vi "ADIS16470 Loop.vi"(8 "error in":errorcluster) -> ()   [LabVIEW 2019]
uses:
  Typedef/ADIS16470 Device Reference.ctl
  Typedef/ADIS16470 Hardware Configuration.ctl
  <vilib>/Rock Robotics/WPI/SPI/WPI_SPIMode.ctl
  <vilib>/Rock Robotics/SystemInterfaces/DIO/FPGA_DIOChannel.ctl
  <vilib>/Rock Robotics/SystemInterfaces/spilib/spi_bus.ctl
  Typedef/ADIS16470 Status.ctl
  Typedef/ADIS16470 Data.ctl
  Typedef/ADIS16470 Process.ctl
  Typedef/ADIS16470 Command Type.ctl
  <vilib>/Rock Robotics/SystemInterfaces/CounterEncoderSourceConvertion/FPGA_CounterEncoderSourceConvertionLVSourceType.ctl
  <vilib>/Rock Robotics/SystemInterfaces/DIO/FPGA_DIODigitalSourceChannel.ctl
  <vilib>/Rock Robotics/SystemInterfaces/AnalogTrigger/FPGA_AnalogTriggerIndex.ctl
  <vilib>/Rock Robotics/SystemInterfaces/AnalogTrigger/FPGA_AnalogTriggerOutType.ctl
  Typedef/ADIS16470 Calibration Time.ctl
  <vilib>/Rock Robotics/WPI/SPI/WPI_SPIDevRef.ctl
  Typedef/ADIS16470 Register.ctl
  <vilib>/Rock Robotics/WPI/Counter/WPI_CounterDigitalInputToDigitalSource.vi
panel:
  in  "Calibration Time":T1
  in  "element":T2
  out "Waveform Chart":dbl(graph)
  out "Offset Bias":i16[](array[numeric])
  in  "ADIS16470DevRef":T3={"DevStatus"={"status"=FALSE, "code"=0, "source"=""}, "Hardware Config"={"SPI Clock Rate (Hz)"=1000000.0, "IMU SPI Mode (3)"=enum."Mode 3 (Clk Idle High,Sample on Trailing)", "IMU Reset Pin"=enum."SPI Port CS2", "IMU SPI Bus"=enum."SPI On-Board, CS0", "IMU Data Ready Pin"=enum."SPI Port CS1", "Stall Config"={"Pow2BytesPerRead"=255, "StallTicks"=640, "CsToSclkTicks"=5}}, "Calibration Complete"=refnum, "Status FIFO"=refnum, "Last Value Reference"=refnum, "Sychronous Process VI"=refnum, "Cmd FIFO"=refnum, "Source"={"DevStatus"={"status"=FALSE, "code"=0, "source"=""}, "AnalogTriggerMode?"=FALSE, "DigitalMode"={"DIO Channel"=enum."Disabled"}, "AnalogTriggerMode"={"AnalogTriggerIndex"=enum."Trig 0", "OutputType"=enum."InWindow"}}, "Data FIFO"=refnum, "Calibration Time"=enum."1s"}
  in  "Main Name":string
  # "XG_BIAS_LOW"
  # "XG_BIAS_HIGH"
  # "YG_BIAS_LOW"
  # "YG_BIAS_HIGH"
  # "ZG_BIAS_LOW"
  # "ZG_BIAS_HIGH"
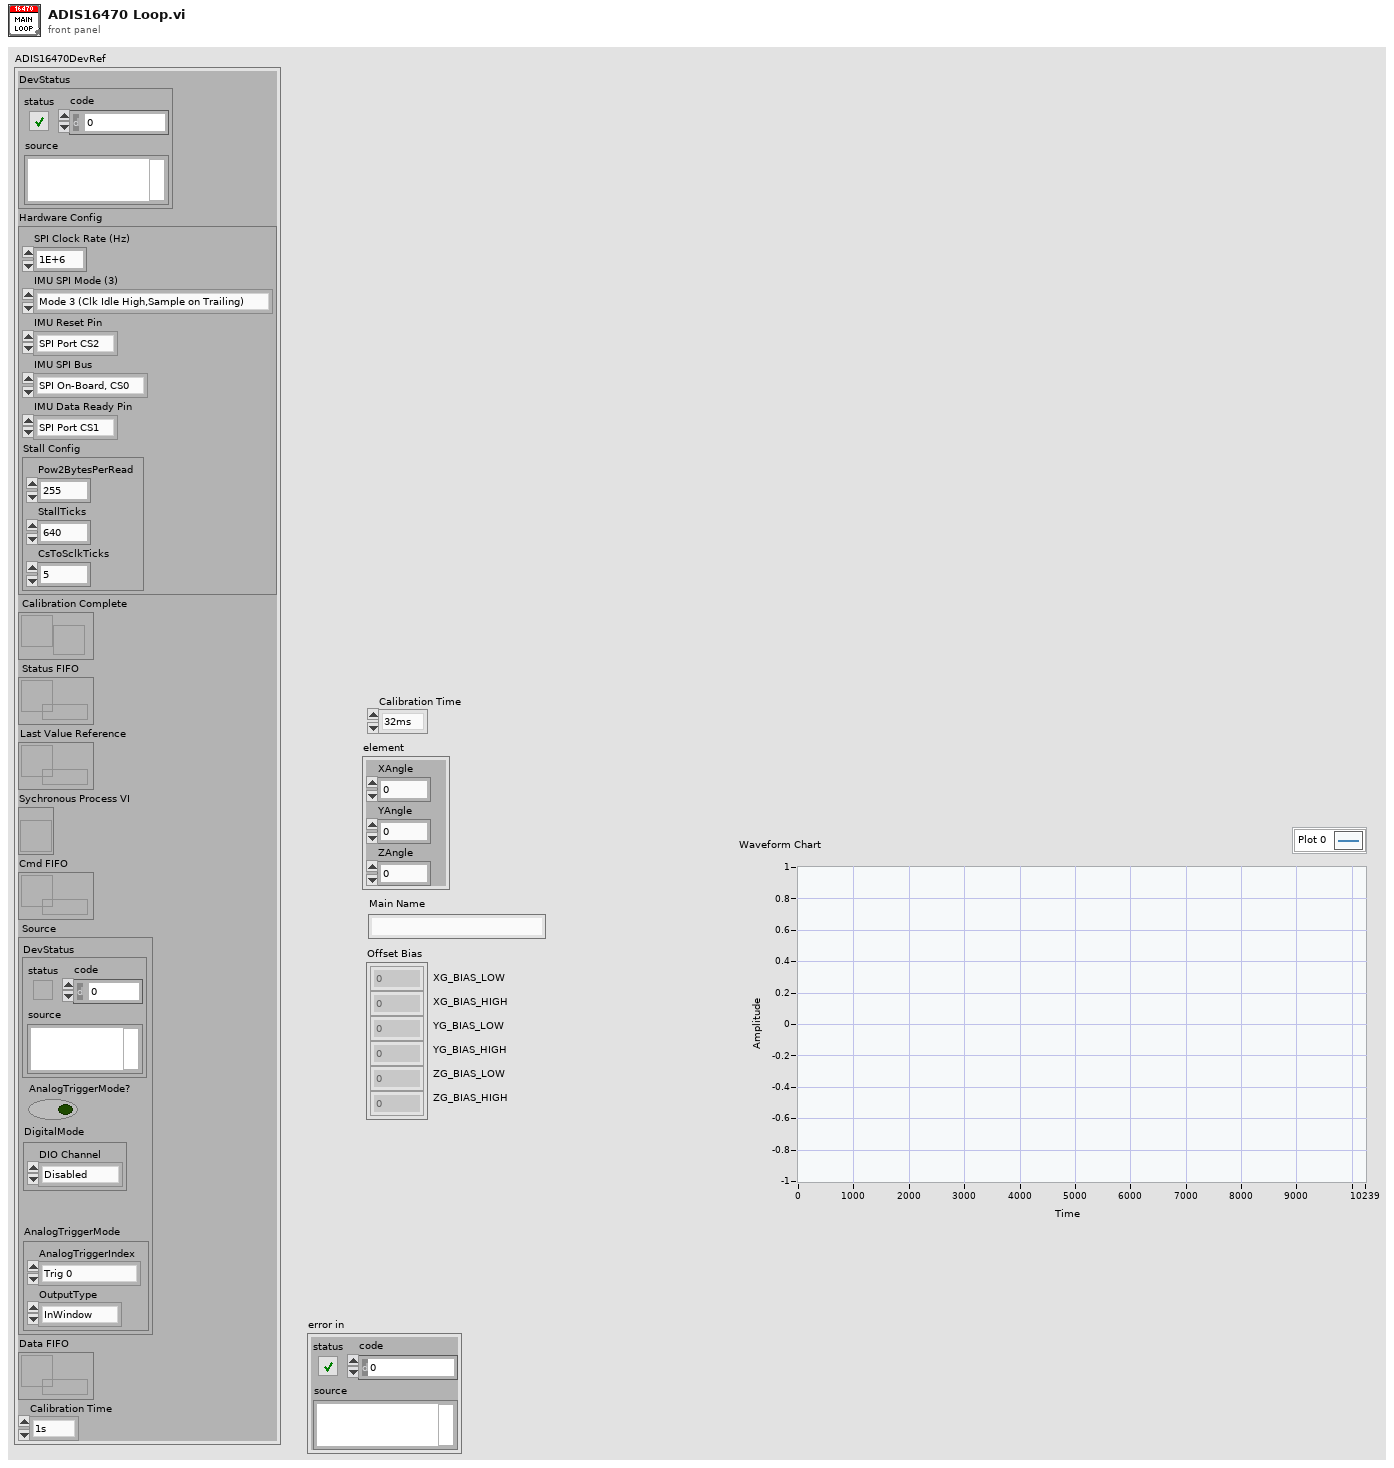
[diagram p1: front panel]
types:
  T1 = typedef "ADIS16470 Calibration Time.ctl" = enum16{"32ms", "64ms", "128ms", "256ms", "512ms", "1s", "2s", "4s", "8s", "16s", "32s", "64s"}
  T2 = typedef "ADIS16470 Data.ctl" = cluster{"XAngle":dbl, "YAngle":dbl, "ZAngle":dbl}
  T3 = typedef "ADIS16470 Device Reference.ctl" = cluster{"DevStatus":errorcluster, "Hardware Config":T4, "Calibration Complete":refnum<notifier>, "Status FIFO":refnum<k33>, "Last Value Reference":refnum<data-value>, "Sychronous Process VI":T8, "Cmd FIFO":refnum<k33>, "Source":T9, "Data FIFO":refnum<k33>, "Calibration Time":T1}
  T4 = typedef "ADIS16470 Hardware Configuration.ctl" = cluster{"SPI Clock Rate (Hz)":dbl, "IMU SPI Mode (3)":T5, "IMU Reset Pin":T6, "IMU SPI Bus":T7, "IMU Data Ready Pin":T6, "Stall Config":cluster{"Pow2BytesPerRead":u8, "StallTicks":u16, "CsToSclkTicks":u8}}
  T5 = typedef "WPI_SPIMode.ctl" = enum16{"Mode 0 (Clk Idle Low,Sample on Leading)", "Mode 1 (Clk Idle Low,Sample on Trailing)", "Mode 2 (Clk Idle High,Sample on Leading)", "Mode 3 (Clk Idle High,Sample on Trailing)"}
  T6 = typedef "FPGA_DIOChannel.ctl" = enum8{"DIO 0", "DIO 1", "DIO 2", "DIO 3", "DIO 4", "DIO 5", "DIO 6", "DIO 7", "DIO 8", "DIO 9", "DIO MXP 0", "DIO MXP 1", "DIO MXP 2", "DIO MXP 3", "DIO MXP 4", "DIO MXP 5", "DIO MXP 6", "DIO MXP 7", "DIO MXP 8", "DIO MXP 9", "DIO MXP 10", "DIO MXP 11", "DIO MXP 12", "DIO MXP 13", "DIO MXP 14", "DIO MXP 15", "SPI Port CS1", "SPI Port CS2", "SPI Port CS3", "SPI Port MISO", "SPI Port MOSI", "Invalid"}
  T7 = typedef "spi_bus.ctl" = enum16{"SPI On-Board, CS0", "SPI On-Board, CS1", "SPI On-Board, CS2", "SPI On-Board, CS3", "SPI MXP", "Invalid"}
  T8 = typedef "ADIS16470 Process.ctl" = refnum<vi>
  T9 = typedef "FPGA_CounterEncoderSourceConvertionLVSourceType.ctl" = cluster{"DevStatus":errorcluster, "AnalogTriggerMode?":bool, "DigitalMode":cluster{"DIO Channel":T10}, "AnalogTriggerMode":cluster{"AnalogTriggerIndex":T11, "OutputType":T12}}
  T10 = typedef "FPGA_DIODigitalSourceChannel.ctl" = enum8{"DIO 0", "DIO 1", "DIO 2", "DIO 3", "DIO 4", "DIO 5", "DIO 6", "DIO 7", "DIO 8", "DIO 9", "DIO MXP 0", "DIO MXP 1", "DIO MXP 2", "DIO MXP 3", "DIO MXP 4", "DIO MXP 5", "DIO MXP 6", "DIO MXP 7", "DIO MXP 8", "DIO MXP 9", "DIO MXP 10", "DIO MXP 11", "DIO MXP 12", "DIO MXP 13", "DIO MXP 14", "DIO MXP 15", "SPI Port CS1", "SPI Port CS2", "SPI Port CS3", "SPI Port MISO", "SPI Port MOSI", "Disabled"}
  T11 = typedef "FPGA_AnalogTriggerIndex.ctl" = enum8{"Trig 0", "Trig 1", "Trig 2", "Trig 3", "Trig 4", "Trig 5", "Trig 6", "Trig 7", "Invalid"}
  T12 = typedef "FPGA_AnalogTriggerOutType.ctl" = enum16{"InWindow", "TriggerState", "Rising", "Falling"}
  T13 = typedef "WPI_SPIDevRef.ctl" = cluster{"DevStatus":errorcluster, "Handle":i32, "SPI Bus":T7}
  T14 = typedef "ADIS16470 Register.ctl" = u8
  T15 = cluster{"SPIDevRef":T13, "Data Counter":u16, "Reset":bool, "Digital Source":T9, "Bytes Per Sample":u32, "Data":dbl[], "ADIS16470DevRef":T3, "TimeStampPrev":u32, "Sensor to Robot Rotation":dbl[][], "Data Packet":T14[], "AutoSPI Active?":bool}
  T16 = typedef "ADIS16470 Status.ctl" = cluster{"Calibrated?":bool, "IMU Detected?":bool}
  T17 = typedef "ADIS16470 Command Type.ctl" = cluster{"Command":enum16{"None", "Reset", "Set Calibration Period", "Recalibrate", "Recal Complete", "Exit Auto SPI", "Start Auto SPI"}, "Data":u32}
  T18 = typedef "WPI_DigitalOutputDevRef.ctl" = cluster{"DIO Channel":T6, "DevStatus":errorcluster}
  T19 = typedef "WPI_DigitalInputDevRef.ctl" = cluster{"DevStatus":errorcluster, "DIO Channel":T6}
  T20 = cluster{"Pow2BytesPerRead":u8, "StallTicks":u16, "CsToSclkTicks":u8}
  T21 = enum16{"None", "Reset", "Set Calibration Period", "Recalibrate", "Recal Complete", "Exit Auto SPI", "Start Auto SPI"}
  T22 = enum32{"Bad", "Idle", "Run top level", "Running"}
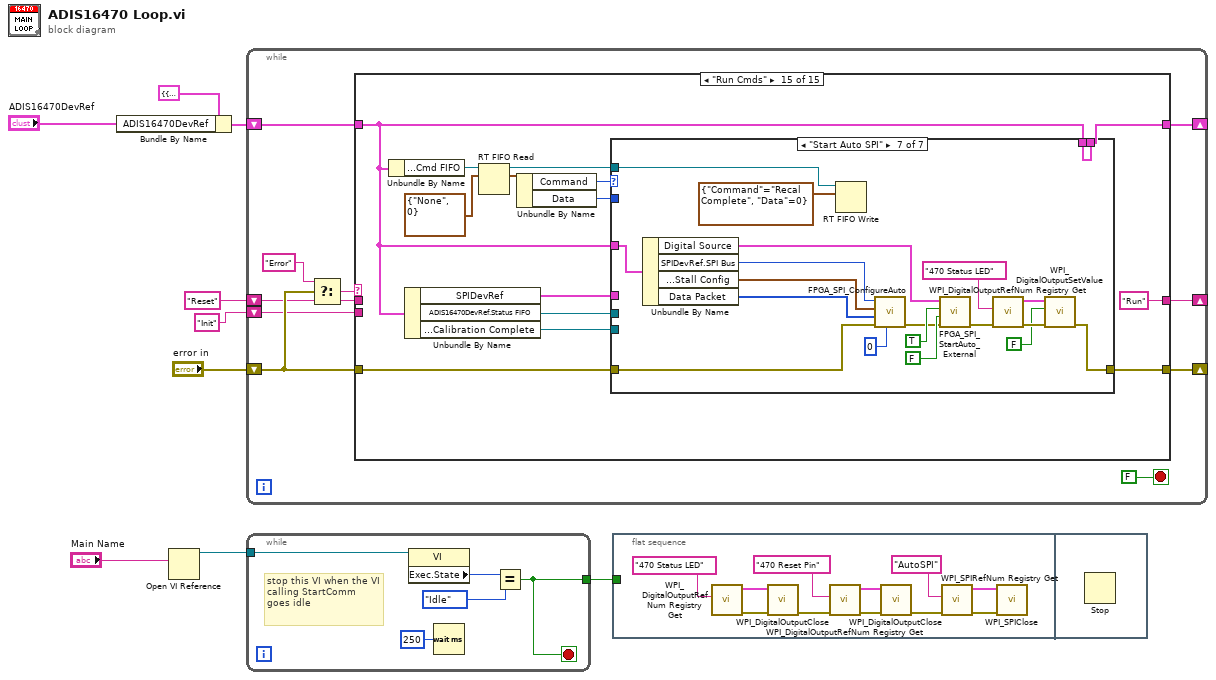
[diagram p0: block diagram]
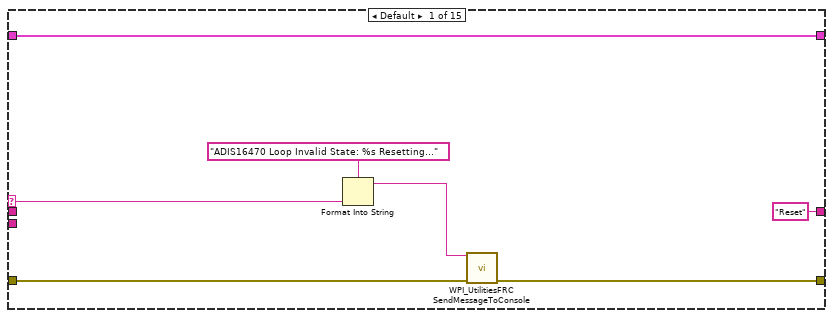
[diagram p2: hidden frame]
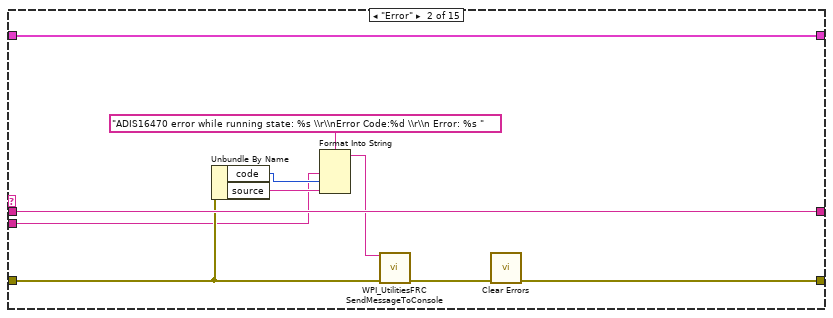
[diagram p3: hidden frame]
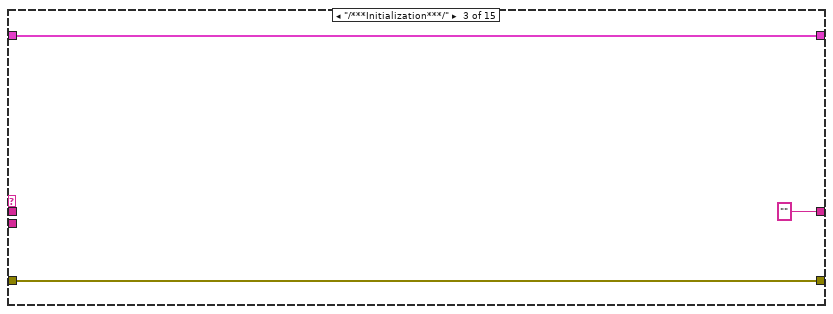
[diagram p4: hidden frame]
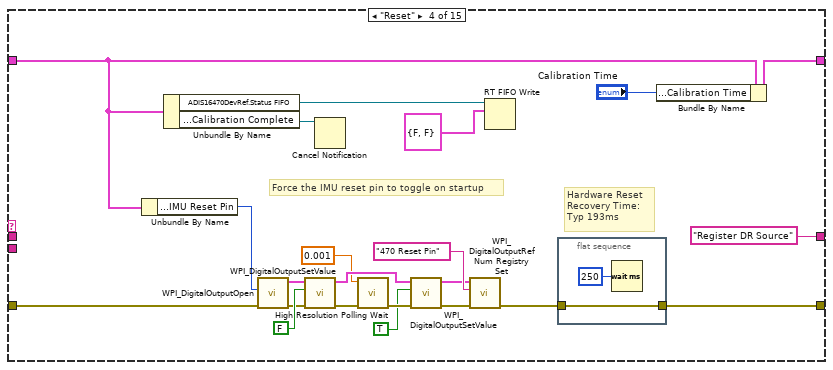
[diagram p5: hidden frame]
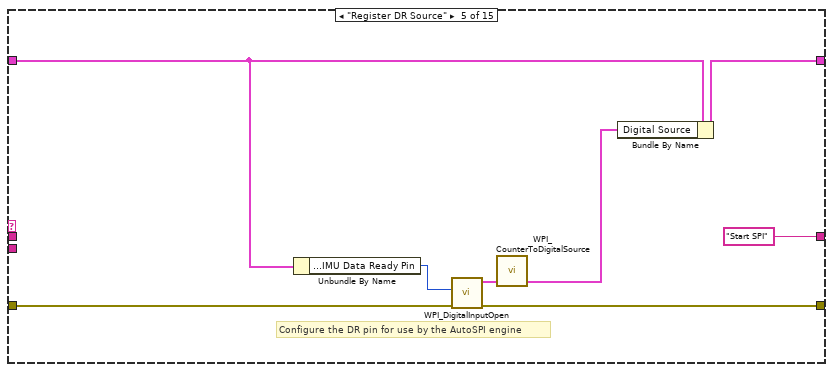
[diagram p6: hidden frame]
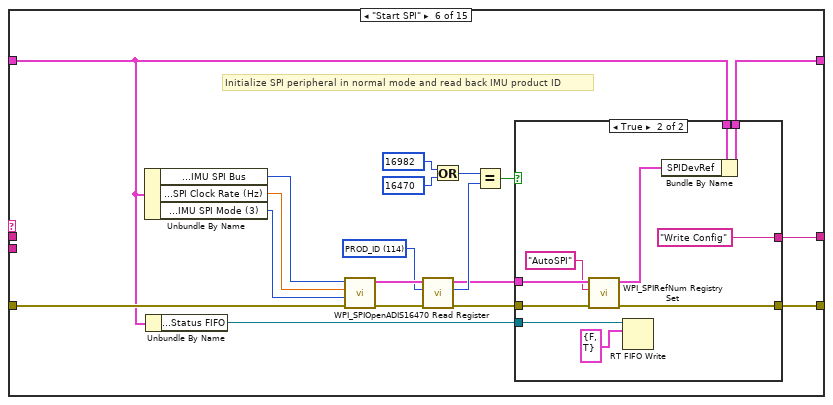
[diagram p7: hidden frame]
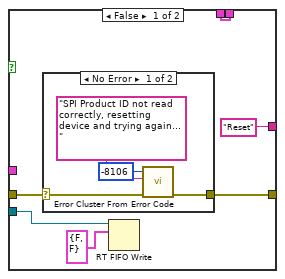
[diagram p8: hidden frame]
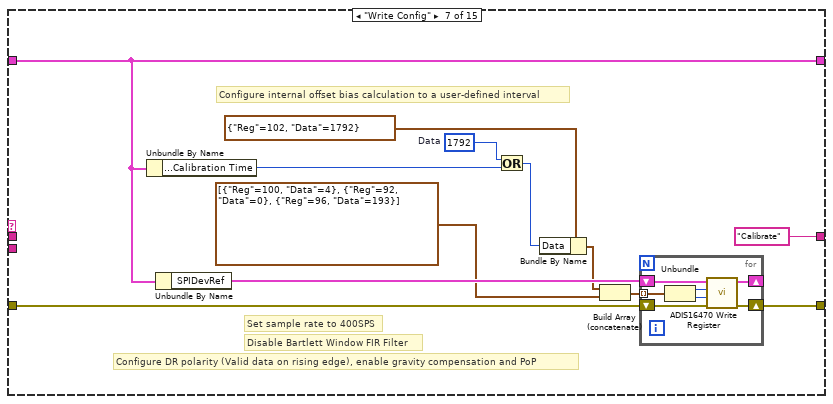
[diagram p10: hidden frame]
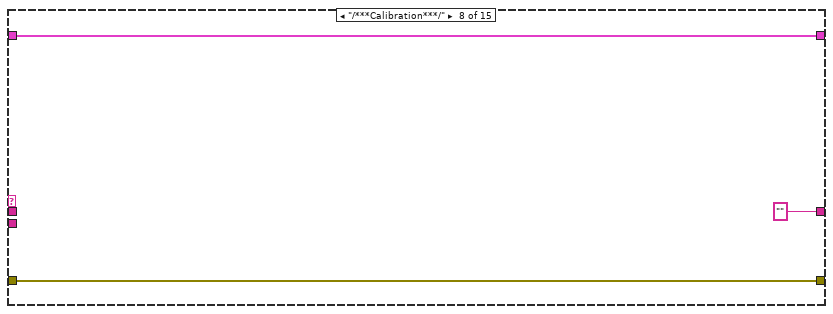
[diagram p11: hidden frame]
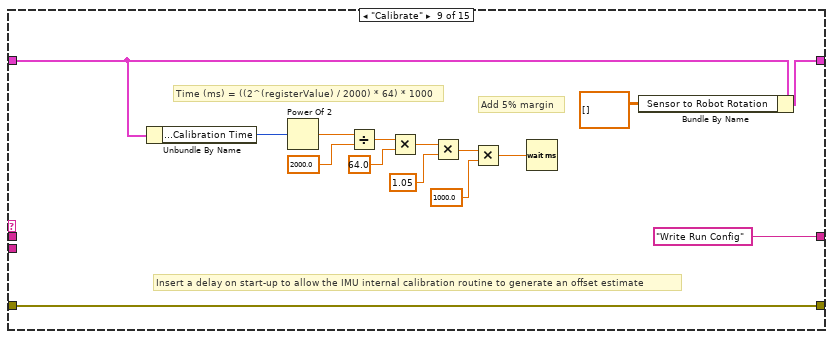
[diagram p12: hidden frame]
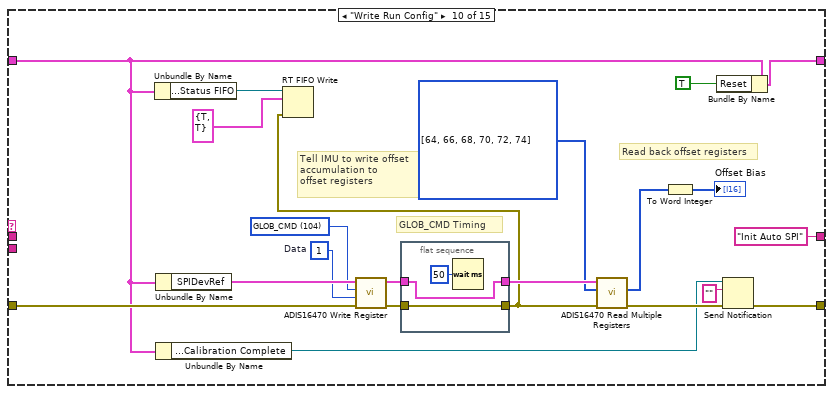
[diagram p13: hidden frame]
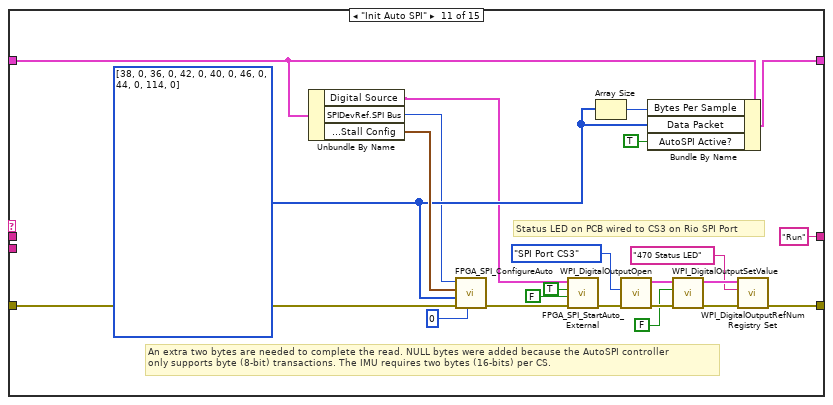
[diagram p14: hidden frame]
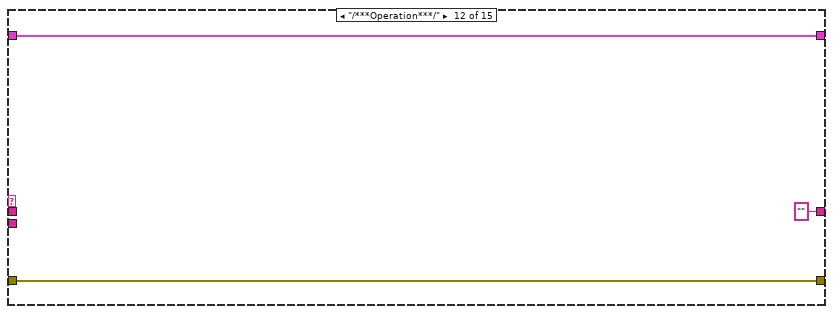
[diagram p15: hidden frame]
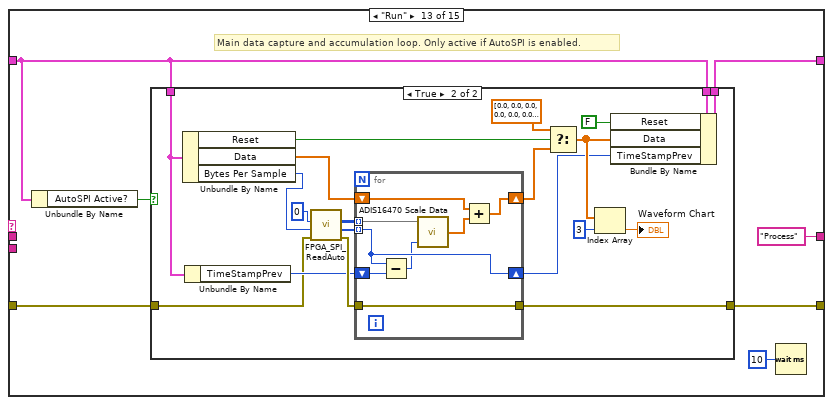
[diagram p16: hidden frame]
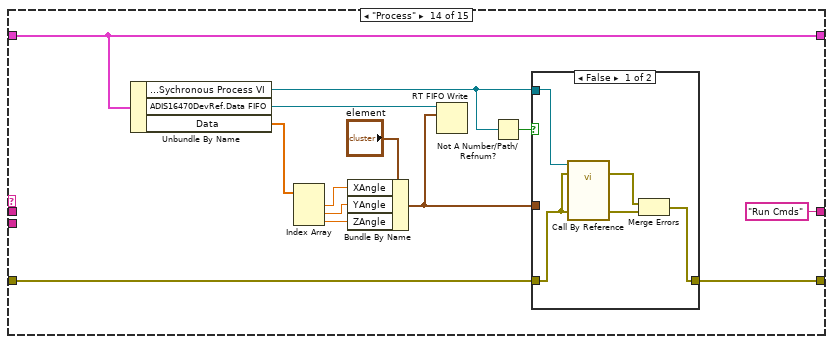
[diagram p18: hidden frame]
diagram:
  n1 = Bundle By Name(cluster=T15 {"SPIDevRef"={"DevStatus"={"status"=FALSE, "code"=0, "source"=""}, "Handle"=0, "SPI Bus"=enum."SPI On-Board, CS0"}, "Data Counter"=0, "Reset"=FALSE, "Digital Source"={"DevStatus"={"status"=FALSE, "code"=0, "source"=""}, "AnalogTriggerMode?"=FALSE, "DigitalMode"={"DIO Channel"=enum."DIO 1"}, "AnalogTriggerMode"={"AnalogTriggerIndex"=enum."Trig 0", "OutputType"=enum."InWindow"}}, "Bytes Per Sample"=0, "Data"=[0.0, 0.0, 0.0, 0.0, 0.0, 0.0, 0.0, 0.0], "ADIS16470DevRef"={"DevStatus"={"status"=FALSE, "code"=0, "source"=""}, "Hardware Config"={"SPI Clock Rate (Hz)"=1000000.0, "IMU SPI Mode (3)"=enum."Mode 3 (Clk Idle High,Sample on Trailing)", "IMU Reset Pin"=enum."SPI Port CS2", "IMU SPI Bus"=enum."SPI On-Board, CS0", "IMU Data Ready Pin"=enum."SPI Port CS1", "Stall Config"={"Pow2BytesPerRead"=255, "StallTicks"=640, "CsToSclkTicks"=5}}, "Calibration Complete"=refnum, "Status FIFO"=refnum, "Last Value Reference"=refnum, "Sychronous Process VI"=refnum, "Cmd FIFO"=refnum, "Source"={"DevStatus"={"status"=FALSE, "code"=0, "source"=""}, "AnalogTriggerMode?"=FALSE, "DigitalMode"={"DIO Channel"=enum."Disabled"}, "AnalogTriggerMode"={"AnalogTriggerIndex"=enum."Trig 0", "OutputType"=enum."InWindow"}}, "Data FIFO"=refnum, "Calibration Time"=enum."1s"}, "TimeStampPrev"=0, "Sensor to Robot Rotation"=[], "Data Packet"=[38, 0, 36, 0, 42, 0, 40, 0, 46, 0, 44, 0, 114, 0], "AutoSPI Active?"=TRUE}, "ADIS16470DevRef"="ADIS16470DevRef") -> (w5:T15)
  n2 = Open VI Reference(vi path="Main Name") -> (vi reference=w8:refnum<vi>)  [unwired: 3 in, 3 out]
  n3 = while {
    shift-right: [w15] -> _
    shift-left: "Reset" -> [w12]
    shift-right: [w17] -> _
    shift-left: w5 -> [w18]
    shift-right: [w16] -> _
    shift-left: "error in" -> [w14]
    shift-left: "Init" -> [w10]
    stop <- FALSE stop-if-true
    n4 = Select(t="Error", s=w14, f=w12) -> (s? t:f=w13:string)
    n5 = case shown="\"Run Cmds\"" w13 {
      selector: w13 -> [w25 _ _ _ _ _ _ _ _ _ _ _ _ _ _]
      tunnel: w18 -> [w26 w36 w39 w42 w67 w73 w113 w133 w144 w154 w187 w198 w200 w247 w256]
      tunnel: [w26 w36 w39 w41 w70 w81 w113 w133 w147 w161 w186 w198 w204 w247 w264] -> w17
      tunnel: w14 -> [w24 w32 w38 w59 w69 w87 w121 w132 w146 w167 w194 w197 w203 w245 w266]
      tunnel: [w23 w33 w38 w57 w64 w80 w120 w132 w146 w156 w178 w197 w202 w244 w265] -> w16
      tunnel: ["Reset" w35 "" "Register DR Source" "Start SPI" w82 "Calibrate" "" "Write Run Config" "Init Auto SPI" "Run" "" "Process" "Run Cmds" "Run"] -> w15
      tunnel: w12 -> [_ w35 _ _ _ _ _ _ _ _ _ _ _ _ _]
      tunnel: w10 -> [_ w27 _ _ _ _ _ _ _ _ _ _ _ _ _]
      frame Default {
        n6 = Format Into String(format string="ADIS16470 Loop Invalid State: %s Resetting...", w25) -> (resulting string=w22:string)  [unwired: 2 in, 1 out]
        n7 = call <vilib>:"WPI_UtilitiesFRC SendMessageToConsole.vi"("Message"=w22, "error in (no error)"=w24) -> ("error out"=w23:errorcluster)  [unwired: 13 in]
      }
      frame "Error" {
        n8 = Unbundle By Name(w32) -> ("code"=w29:i32, "source"=w28:string)
        n9 = Format Into String(format string="ADIS16470 error while running state: %s \\r\\nError Code:%d \\r\\n Error: %s ", w27, w29, w28) -> (resulting string=w31:string)  [unwired: 2 in, 1 out]
        n10 = call <vilib>:"WPI_UtilitiesFRC SendMessageToConsole.vi"("Message"=w31, "error in (no error)"=w32) -> ("error out"=w34:errorcluster)  [unwired: 13 in]
        n11 = call <vilib>:"Clear Errors.vi"("error in (no error)"=w34) -> ("error out"=w33:errorcluster)  [unwired: 5 in, 1 out]
      }
      frame "/***Initialization***/" {
      }
      frame "Reset" {
        # "Hardware Reset Recovery Time: Typ 193ms"
        # "Force the IMU reset pin to toggle on startup"
        n12 = Unbundle By Name(w42) -> ("ADIS16470DevRef.Hardware Config.IMU Reset Pin"=w60:T6)
        n13 = Unbundle By Name(w42) -> ("ADIS16470DevRef.Status FIFO"=w55:refnum<k33>, "ADIS16470DevRef.Calibration Complete"=w56:refnum<notifier>)
        n14 = call <vilib>:"WPI_DigitalOutputOpen.vi"("error in (no error)"=w59, "DIO Channel"=w60) -> ("error out"=w52:errorcluster, "DigitalOutputDevRef"=w61:T18)  [unwired: 8 in]
        n15 = call <vilib>:"WPI_DigitalOutputSetValue.vi"("error in (no error)"=w52, "Value"=FALSE, "DigitalOutputDevRef"=w61) -> ("error out"=w49:errorcluster, "DigitalOutputDevRef"=w47:T18)  [unwired: 7 in]
        n16 = Cancel Notification(0:w56) -> ()  [unwired: 1 in, 3 out]
        n17 = call <vilib>:"High Resolution Polling Wait.vi"("error in (no error)"=w49, "seconds to wait"=0.001) -> ("error out"=w48:errorcluster)  [unwired: 9 in]
        n18 = call <vilib>:"WPI_DigitalOutputSetValue.vi"("error in (no error)"=w48, "Value"=TRUE, "DigitalOutputDevRef"=w47) -> ("error out"=w44:errorcluster, "DigitalOutputDevRef"=w45:T18)  [unwired: 7 in]
        n19 = call <vilib>:"WPI_DigitalOutputRefNum Registry Set.vi"("error in (no error)"=w44, "refnum name"="470 Reset Pin", "DigitalOutputDevRef"=w45) -> ("error out"=w50:errorcluster)  [unwired: 7 in, 1 out]
        n20 = RT FIFO Write(0:w55, 1:T16 {"Calibrated?"=FALSE, "IMU Detected?"=FALSE} ("element")) -> ()  [unwired: 3 in, 4 out]
        n21 = flat-sequence {
          tunnel: [w63] -> w57
          tunnel: w50 -> [w63]
          frame #0 {
            n22 = Wait (ms)(milliseconds to wait=u32 250) -> ()  [unwired: 1 out]
          }
        }
        n23 = Bundle By Name(cluster=w42, "ADIS16470DevRef.Calibration Time"="Calibration Time") -> (w41:T15)
      }
      frame "Register DR Source" {
        # "Configure the DR pin for use by the AutoSPI engine"
        n24 = Unbundle By Name(w67) -> ("ADIS16470DevRef.Hardware Config.IMU Data Ready Pin"=w66:T6)
        n25 = call <vilib>:"WPI_DigitalInputOpen.vi"("error in (no error)"=w69, "DIO Channel"=w66) -> ("error out"=w64:errorcluster, "DigitalInputDevRef"=w68:T19)  [unwired: 8 in]
        n26 = call-poly <vilib>:"WPI_CounterToDigitalSource.vi"("DigitalInputDevRef"=w68) -> ("Digital Source"=w65:T9)  [unwired: 6 in]
        n27 = Bundle By Name(cluster=w67, "Digital Source"=w65) -> (w70:T15)
      }
      frame "Start SPI" {
        w75 = T14 114 items=["Reserved1"=0, "DIAG_STAT"=2, "X_GYRO_LOW"=4, "X_GYRO_OUT"=6, "Y_GYRO_LOW"=8, "Y_GYRO_OUT"=10, "Z_GYRO_LOW"=12, "Z_GYRO_OUT"=14, "X_ACCL_LOW"=16, "X_ACCL_OUT"=18, "Y_ACCL_LOW"=20, "Y_ACCL_OUT"=22, "Z_ACCL_LOW"=24, "Z_ACCL_OUT"=26, "TEMP_OUT"=28, "TIME_STAMP"=30, "Reseved2"=32, "DATA_CNTR"=34, "X_DELTANG_LOW"=36, "X_DELTANG_OUT"=38, "Y_DELTANG_LOW"=40, "Y_DELTANG_OUT"=42, "Z_DELTANG_LOW"=44, "Z_DELTANG_OUT"=46, "X_DELTVEL_LOW"=48, "X_DELTVEL_OUT"=50, "Y_DELTVEL_LOW"=52, "Y_DELTVEL_OUT"=54, "Z_DELTVEL_LOW"=56, "Z_DELTVEL_OUT"=58, "Reserved3"=60, "Reserved4"=62, "XG_BIAS_LOW"=64, "XG_BIAS_HIGH"=66, "YG_BIAS_LOW"=68, "YG_BIAS_OUT"=70, "ZG_BIAS_LOW"=72, "ZG_BIAS_OUT"=74, "XA_BIAS_LOW"=76, "XA_BIAS_HIGH"=78, "YA_BIAS_LOW"=80, "YA_BIAS_OUT"=82, "ZA_BIAS_LOW"=84, "ZA_BIAS_OUT"=86, "Reserved5"=88, "Reserved6"=90, "FILT_CTRL"=92, "Reserved5"=94, "MSC_CTRL"=96, "UP_SCALE"=98, "DEC_RATE"=100, "NULL_CNFG"=102, "GLOB_CMD"=104, "Reserved6"=106, "FIRM_REV"=108, "FIRM_DM"=110, "FIRM_Y"=112, "PROD_ID"=114, "SERIAL_NUM"=116, "USER_SCR1"=118, "USER_SCR2"=120, "USER_SCR3"=122, "FLSHCNT_LOW"=124, "FLSHCNT_HIGH"=126] ("ADIS16448 Register")
        # "Initialize SPI peripheral in normal mode and read back IMU product ID"
        n28 = Unbundle By Name(w73) -> ("ADIS16470DevRef.Hardware Config.IMU SPI Bus"=w83:T7, "ADIS16470DevRef.Hardware Config.SPI Clock Rate (Hz)"=w84:dbl, "ADIS16470DevRef.Hardware Config.IMU SPI Mode (3)"=w85:T5)
        n29 = Unbundle By Name(w73) -> ("ADIS16470DevRef.Status FIFO"=w72:refnum<k33>)
        n30 = call <vilib>:"WPI_SPIOpen.vi"("error in"=w87, "Mode (3)"=w85, "Clock Rate (Hz)"=w84, "SPI Bus"=w83) -> ("error out"=w77:errorcluster, "SPIDevRef"=w76:T13)  [unwired: 6 in]
        n31 = call "ADIS16470 Read Register.vi"("error in (no error)"=w77, "ADIS16470 Register"=w75, "SPIDevRef in"=w76) -> ("error out"=w78:errorcluster, "Register Value"=w79:u16, "SPIDevRef out"=w74:T13)  [unwired: 6 in]
        n32 = Or(x=u16 16982 ("y"), y=u16 16470) -> (x .or. y?=w88:u16)
        n33 = Equal?(x=w88, y=w79) -> (x = y?=w86:bool)
        n34 = case shown="True" w86 {
          tunnel: ["Reset" "Write Config"] -> w82
          tunnel: w73 -> [w95 w110]
          tunnel: [w95 w109] -> w81
          tunnel: [w94 w105] -> w80
          tunnel: w78 -> [w93 w108]
          tunnel: w74 -> [_ w107]
          tunnel: w72 -> [w91 w103]
          frame False {
            n35 = case shown="No Error" w93 {
              selector: w93 -> [w99 w101]
              tunnel: [w100 w101] -> w94
              frame No Error {
                n36 = call <vilib>:"Error Cluster From Error Code.vi"("error in (no error)"=w99, "error message (\"\")"="SPI Product ID not read correctly, resetting device and trying again..." ("error message (\"\")"), "error code (0)"=-8106) -> ("error out"=w100:errorcluster)  [unwired: 6 in]
              }
              frame Error {
              }
            }
            n37 = RT FIFO Write(0:w91, 1:T16 {"Calibrated?"=FALSE, "IMU Detected?"=FALSE} ("element")) -> ()  [unwired: 3 in, 4 out]
          }
          frame True {
            n38 = call <vilib>:"WPI_SPIRefNum Registry Set.vi"("error in (no error)"=w108, "refnum name"="AutoSPI", "SPIDevRef"=w107) -> ("error out"=w105:errorcluster, "SPIDevRef"=w106:T13)  [unwired: 7 in]
            n39 = RT FIFO Write(0:w103, 1:T16 {"Calibrated?"=FALSE, "IMU Detected?"=TRUE} ("element")) -> ()  [unwired: 3 in, 4 out]
            n40 = Bundle By Name(cluster=w110, "SPIDevRef"=w106) -> (w109:T15)
          }
        }
      }
      frame "Write Config" {
        w115 = 1792  # Data
        # "Set sample rate to 400SPS"
        # "Configure internal offset bias calculation to a user-defined interval"
        # "Configure DR polarity (Valid data on rising edge), enable gravity compensation and PoP"
        # "Disable Bartlett Window FIR Filter"
        n41 = Unbundle By Name(w113) -> ("ADIS16470DevRef.Calibration Time"=w112:T1)
        n42 = Unbundle By Name(w113) -> ("SPIDevRef"=w122:T13)
        n43 = Or(x=w115, y=w112) -> (x .or. y?=w114:i32)
        n44 = Bundle By Name(cluster=cluster{"Reg":T14, "Data":i32} {"Reg"=102, "Data"=1792}, "Data"=w114) -> (w116:cluster{"Reg":T14, "Data":i32})
        n45 = Build Array (concatenate)(w116, cluster{"Reg":T14, "Data":u16}[] [{"Reg"=100, "Data"=4}, {"Reg"=92, "Data"=0}, {"Reg"=96, "Data"=193}]) -> (w117:cluster{"Reg":T14, "Data":i32}[])
        n46 = for {
          tunnel: w117 -> [w130] mode=indexing
          shift-right: [w126] -> w120
          shift-left: w121 -> [w125]
          shift-right: [w124] -> _
          shift-left: w122 -> [w127]
          n47 = Unbundle(w130) -> ("Reg"=w129:T14, "Data"=w128:i32)
          n48 = call "ADIS16470 Write Register.vi"("error in (no error)"=w125, "Data"=w128, "Register"=w129, "SPIDevRef in"=w127) -> ("error out"=w126:errorcluster, "SPIDevRef out"=w124:T13)  [unwired: 6 in]
        }
      }
      frame "/***Calibration***/" {
      }
      frame "Calibrate" {
        # "Insert a delay on start-up to allow the IMU internal calibration routine to generate an offset estimate"
        # "Add 5% margin"
        # "Time (ms) = ((2^(registerValue) / 2000) * 64) * 1000"
        n49 = Unbundle By Name(w144) -> ("ADIS16470DevRef.Calibration Time"=w143:T1)
        n50 = Power Of 2(x=w143) -> (2^x=w142:dbl)
        n51 = Divide(x=w142, y=2000.0) -> (x/y=w140:dbl)
        n52 = Multiply(x=w140, y=64.0) -> (x*y=w138:dbl)
        n53 = Multiply(x=w138, y=1.05) -> (x*y=w136:dbl)
        n54 = Multiply(x=w136, y=1000.0) -> (x*y=w134:dbl)
        n55 = Wait (ms)(milliseconds to wait=w134) -> ()  [unwired: 1 out]
        n56 = Bundle By Name(cluster=w144, "Sensor to Robot Rotation"=dbl[][] []) -> (w147:T15)
      }
      frame "Write Run Config" {
        w151 = T14 104 items=["Reserved1"=0, "DIAG_STAT"=2, "X_GYRO_LOW"=4, "X_GYRO_OUT"=6, "Y_GYRO_LOW"=8, "Y_GYRO_OUT"=10, "Z_GYRO_LOW"=12, "Z_GYRO_OUT"=14, "X_ACCL_LOW"=16, "X_ACCL_OUT"=18, "Y_ACCL_LOW"=20, "Y_ACCL_OUT"=22, "Z_ACCL_LOW"=24, "Z_ACCL_OUT"=26, "TEMP_OUT"=28, "TIME_STAMP"=30, "Reseved2"=32, "DATA_CNTR"=34, "X_DELTANG_LOW"=36, "X_DELTANG_OUT"=38, "Y_DELTANG_LOW"=40, "Y_DELTANG_OUT"=42, "Z_DELTANG_LOW"=44, "Z_DELTANG_OUT"=46, "X_DELTVEL_LOW"=48, "X_DELTVEL_OUT"=50, "Y_DELTVEL_LOW"=52, "Y_DELTVEL_OUT"=54, "Z_DELTVEL_LOW"=56, "Z_DELTVEL_OUT"=58, "Reserved3"=60, "Reserved4"=62, "XG_BIAS_LOW"=64, "XG_BIAS_HIGH"=66, "YG_BIAS_LOW"=68, "YG_BIAS_OUT"=70, "ZG_BIAS_LOW"=72, "ZG_BIAS_OUT"=74, "XA_BIAS_LOW"=76, "XA_BIAS_HIGH"=78, "YA_BIAS_LOW"=80, "YA_BIAS_OUT"=82, "ZA_BIAS_LOW"=84, "ZA_BIAS_OUT"=86, "Reserved5"=88, "Reserved6"=90, "FILT_CTRL"=92, "Reserved5"=94, "MSC_CTRL"=96, "UP_SCALE"=98, "DEC_RATE"=100, "NULL_CNFG"=102, "GLOB_CMD"=104, "Reserved6"=106, "FIRM_REV"=108, "FIRM_DM"=110, "FIRM_Y"=112, "PROD_ID"=114, "SERIAL_NUM"=116, "USER_SCR1"=118, "USER_SCR2"=120, "USER_SCR3"=122, "FLSHCNT_LOW"=124, "FLSHCNT_HIGH"=126] ("Register")
        w166 = u16 1  # Data
        w162 = T14[] [64, 66, 68, 70, 72, 74] items=["Reserved1"=0, "DIAG_STAT"=2, "X_GYRO_LOW"=4, "X_GYRO_OUT"=6, "Y_GYRO_LOW"=8, "Y_GYRO_OUT"=10, "Z_GYRO_LOW"=12, "Z_GYRO_OUT"=14, "X_ACCL_LOW"=16, "X_ACCL_OUT"=18, "Y_ACCL_LOW"=20, "Y_ACCL_OUT"=22, "Z_ACCL_LOW"=24, "Z_ACCL_OUT"=26, "TEMP_OUT"=28, "TIME_STAMP"=30, "Reseved2"=32, "DATA_CNTR"=34, "X_DELTANG_LOW"=36, "X_DELTANG_OUT"=38, "Y_DELTANG_LOW"=40, "Y_DELTANG_OUT"=42, "Z_DELTANG_LOW"=44, "Z_DELTANG_OUT"=46, "X_DELTVEL_LOW"=48, "X_DELTVEL_OUT"=50, "Y_DELTVEL_LOW"=52, "Y_DELTVEL_OUT"=54, "Z_DELTVEL_LOW"=56, "Z_DELTVEL_OUT"=58, "Reserved3"=60, "Reserved4"=62, "XG_BIAS_LOW"=64, "XG_BIAS_HIGH"=66, "YG_BIAS_LOW"=68, "YG_BIAS_HIGH"=70, "ZG_BIAS_LOW"=72, "ZG_BIAS_HIGH"=74, "XA_BIAS_LOW"=76, "XA_BIAS_HIGH"=78, "YA_BIAS_LOW"=80, "YA_BIAS_HIGH"=82, "ZA_BIAS_LOW"=84, "ZA_BIAS_HIGH"=86, "Reserved5"=88, "Reserved6"=90, "FILT_CTRL"=92, "Reserved5"=94, "MSC_CTRL"=96, "UP_SCALE"=98, "DEC_RATE"=100, "NULL_CNFG"=102, "GLOB_CMD"=104, "Reserved6"=106, "FIRM_REV"=108, "FIRM_DM"=110, "FIRM_Y"=112, "PROD_ID"=114, "SERIAL_NUM"=116, "USER_SCR1"=118, "USER_SCR2"=120, "USER_SCR3"=122, "FLSHCNT_LOW"=124, "FLSHCNT_HIGH"=126] ("Registers")
        # "Tell IMU to write offset \naccumulation to \noffset registers"
        # "GLOB_CMD Timing"
        # "Read back offset registers"
        n57 = Unbundle By Name(w154) -> ("ADIS16470DevRef.Status FIFO"=w153:refnum<k33>)
        n58 = Unbundle By Name(w154) -> ("SPIDevRef"=w168:T13)
        n59 = Unbundle By Name(w154) -> ("ADIS16470DevRef.Calibration Complete"=w157:refnum<notifier>)
        n60 = RT FIFO Write(0:w153, 1:T16 {"Calibrated?"=TRUE, "IMU Detected?"=TRUE} ("element"), 3:w150) -> ()  [unwired: 2 in, 4 out]
        n61 = call "ADIS16470 Write Register.vi"("error in (no error)"=w167, "Data"=w166, "Register"=w151, "SPIDevRef in"=w168) -> ("error out"=w165:errorcluster, "SPIDevRef out"=w164:T13)  [unwired: 6 in]
        n62 = flat-sequence {
          tunnel: w165 -> [w172]
          tunnel: [w172] -> w150
          tunnel: w164 -> [w170]
          tunnel: [w170] -> w163
          frame #0 {
            n63 = Wait (ms)(milliseconds to wait=u32 50) -> ()  [unwired: 1 out]
          }
        }
        n64 = call "ADIS16470 Read Multiple Registers.vi"("error in (no error)"=w150, "Registers"=w162, "SPIDevRefIn"=w163) -> ("error out"=w158:errorcluster, "Values"=w149:u16[])  [unwired: 6 in, 1 out]
        n65 = To Word Integer(number=w149) -> (16bit integer=→"Offset Bias":i16[])
        n66 = Bundle By Name(cluster=w154, "Reset"=TRUE ("First Run")) -> (w161:T15)
        n67 = Send Notification(notification="", notifier=w157, error in (no error)=w158) -> (error out=w156:errorcluster)  [unwired: 1 out]
      }
      frame "Init Auto SPI" {
        w175 = T14[] [38, 0, 36, 0, 42, 0, 40, 0, 46, 0, 44, 0, 114, 0] items=["NULL"=0, "DIAG_STAT"=2, "X_GYRO_LOW"=4, "X_GYRO_OUT"=6, "Y_GYRO_LOW"=8, "Y_GYRO_OUT"=10, "Z_GYRO_LOW"=12, "Z_GYRO_OUT"=14, "X_ACCL_LOW"=16, "X_ACCL_OUT"=18, "Y_ACCL_LOW"=20, "Y_ACCL_OUT"=22, "Z_ACCL_LOW"=24, "Z_ACCL_OUT"=26, "TEMP_OUT"=28, "TIME_STAMP"=30, "Reseved2"=32, "DATA_CNTR"=34, "X_DELTANG_LOW"=36, "X_DELTANG_OUT"=38, "Y_DELTANG_LOW"=40, "Y_DELTANG_OUT"=42, "Z_DELTANG_LOW"=44, "Z_DELTANG_OUT"=46, "X_DELTVEL_LOW"=48, "X_DELTVEL_OUT"=50, "Y_DELTVEL_LOW"=52, "Y_DELTVEL_OUT"=54, "Z_DELTVEL_LOW"=56, "Z_DELTVEL_OUT"=58, "Reserved3"=60, "Reserved4"=62, "XG_BIAS_LOW"=64, "XG_BIAS_HIGH"=66, "YG_BIAS_LOW"=68, "YG_BIAS_HIGH"=70, "ZG_BIAS_LOW"=72, "ZG_BIAS_HIGH"=74, "XA_BIAS_LOW"=76, "XA_BIAS_HIGH"=78, "YA_BIAS_LOW"=80, "YA_BIAS_HIGH"=82, "ZA_BIAS_LOW"=84, "ZA_BIAS_HIGH"=86, "Reserved5"=88, "Reserved6"=90, "FILT_CTRL"=92, "Reserved5"=94, "MSC_CTRL"=96, "UP_SCALE"=98, "DEC_RATE"=100, "NULL_CNFG"=102, "GLOB_CMD"=104, "Reserved6"=106, "FIRM_REV"=108, "FIRM_DM"=110, "FIRM_Y"=112, "PROD_ID"=114, "SERIAL_NUM"=116, "USER_SCR1"=118, "USER_SCR2"=120, "USER_SCR3"=122, "FLSHCNT_LOW"=124, "FLSHCNT_HIGH"=126] ("Registers")
        # "Status LED on PCB wired to CS3 on Rio SPI Port"
        # "An extra two bytes are needed to complete the read. NULL bytes were added because the AutoSPI controller \nonly supports byte (8-bit) transactions. The IMU requires two bytes (16-bits) per CS."
        n68 = Unbundle By Name(w187) -> ("Digital Source"=w174:T9, "SPIDevRef.SPI Bus"=w173:T7, "ADIS16470DevRef.Hardware Config.Stall Config"=w177:T20)
        n69 = call <vilib>:"FPGA_SPI_ConfigureAuto.vi"("SPI Auto Zero Byte Count"=u8 0, "error in"=w194, "SPI Auto TX Byte Array"=w175, "Stall Config"=w177, "SPI Bus"=w173) -> ("error out"=w192:errorcluster)  [unwired: 6 in]
        n70 = call <vilib>:"FPGA_SPI_StartAuto_External.vi"("error in (no error)"=w192, "Falling Edge"=FALSE, "Rising Edge"=TRUE, "Source"=w174) -> ("error out"=w188:errorcluster)  [unwired: 7 in]
        n71 = Array Size(array=w175) -> (size(s)=w185:i32)
        n72 = call <vilib>:"WPI_DigitalOutputOpen.vi"("error in (no error)"=w188, "DIO Channel"=FPGA_DIOChannel."SPI Port CS3") -> ("error out"=w184:errorcluster, "DigitalOutputDevRef"=w183:T18)  [unwired: 8 in]
        n73 = Bundle By Name(cluster=w187, "Bytes Per Sample"=w185, "Data Packet"=w175, "AutoSPI Active?"=TRUE) -> (w186:T15)
        n74 = call <vilib>:"WPI_DigitalOutputSetValue.vi"("error in (no error)"=w184, "Value"=FALSE, "DigitalOutputDevRef"=w183) -> ("error out"=w181:errorcluster, "DigitalOutputDevRef"=w180:T18)  [unwired: 7 in]
        n75 = call <vilib>:"WPI_DigitalOutputRefNum Registry Set.vi"("error in (no error)"=w181, "refnum name"="470 Status LED", "DigitalOutputDevRef"=w180) -> ("error out"=w178:errorcluster)  [unwired: 7 in, 1 out]
      }
      frame "/***Operation***/" {
      }
      frame "Run" {
        # "Main data capture and accumulation loop. Only active if AutoSPI is enabled."
        n76 = Unbundle By Name(w200) -> ("AutoSPI Active?"=w199:bool)
        n77 = case shown="True" w199 {
          tunnel: [w207 w227] -> w204
          tunnel: w203 -> [w206 w208]
          tunnel: [w206 w217] -> w202
          tunnel: w200 -> [w207 w212]
          tunnel: w200 -> [_ w209]
          frame False {
          }
          frame True {
            n78 = Unbundle By Name(w209) -> ("Reset"=w225:bool, "Data"=w220:dbl[], "Bytes Per Sample"=w224:u32)
            n79 = Unbundle By Name(w209) -> ("TimeStampPrev"=w211:u32)
            n80 = call <vilib>:"FPGA_SPI_ReadAuto.vi"("error in (no error)"=w208, "Bytes per Sample"=w224, "Samples to Read"=u32 0) -> ("error out"=w218:errorcluster, "Timestamps"=w221:u32[], "Data"=w222:u8[][])  [unwired: 6 in]
            n81 = for {
              tunnel: w222 -> [w229] mode=indexing
              tunnel: w221 -> [w232] mode=indexing
              shift-right: [w235] -> w219
              shift-left: w220 -> [w234]
              tunnel: w218 -> [w231]
              tunnel: [w231] -> w217
              shift-right: [w232] -> w210
              shift-left: w211 -> [w233]
              n82 = Subtract(x=w232, y=w233) -> (x-y=w228:u32)
              n83 = call "ADIS16470 Scale Data.vi"("TimeStamp"=w228, "Data In"=w229) -> ("Scaled Data Out"=w230:dbl[])  [unwired: 3 in]
              n84 = Add(x=w234, y=w230) -> (x+y=w235:dbl[])
            }
            n85 = Select(t=dbl[] [0.0, 0.0, 0.0, 0.0, 0.0, 0.0, 0.0, 0.0] ("Angle and Vel"), s=w225, f=w219) -> (s? t:f=w215:dbl[])
            n86 = Index Array(array=w215, index=3) -> (element=→"Waveform Chart":dbl)
            n87 = Bundle By Name(cluster=w212, "Reset"=FALSE ("First Run"), "Data"=w215, "TimeStampPrev"=w210) -> (w227:T15)
          }
        }
        n88 = Wait (ms)(milliseconds to wait=u32 10) -> ()  [unwired: 1 out]
      }
      frame "Process" {
        n89 = Unbundle By Name(w247) -> ("ADIS16470DevRef.Sychronous Process VI"=w242:T8, "ADIS16470DevRef.Data FIFO"=w246:refnum<k33>, "Data"=w241:dbl[])
        n90 = Index Array(array=w241) -> (element #1=w240:dbl, element #2=w239:dbl, element #3=w238:dbl)  [unwired: 3 in]
        n91 = Bundle By Name(cluster="element", "XAngle"=w240, "YAngle"=w239, "ZAngle"=w238) -> (w236:T2)
        n92 = RT FIFO Write(0:w246, 1:w236) -> ()  [unwired: 3 in, 4 out]
        n93 = Not A Number/Path/Refnum?(number/path/refnum=w242) -> (NaN/Path/Refnum?=w243:bool)
        n94 = case shown="False" w243 {
          tunnel: w245 -> [w249 w254]
          tunnel: w236 -> [_ _]
          tunnel: [w253 w254] -> w244
          tunnel: w242 -> [w252 _]
          frame False {
            n95 = call-by-ref "?"(reference=w252, error in=w249, 8:"error in (no error)"=w249) -> (error out=w250:errorcluster, 0:"error out"=w251:errorcluster)  [unwired: 10 in, 1 out]
            n96 = Merge Errors(w250, w251) -> (w253:errorcluster)
          }
          frame True {
          }
        }
      }
      frame "Run Cmds" {
        n97 = Unbundle By Name(w256) -> ("ADIS16470DevRef.Cmd FIFO"=w267:refnum<k33>)
        n98 = Unbundle By Name(w256) -> ("SPIDevRef"=w255:T13, "ADIS16470DevRef.Status FIFO"=w262:refnum<k33>, "ADIS16470DevRef.Calibration Complete"=w263:refnum<notifier>)
        n99 = RT FIFO Read(0:w267, 1:T17 {"Command"=enum."None", "Data"=0} ("element")) -> (8:w260:refnum<k33>, 9:w259:T17)  [unwired: 2 in, 3 out]
        n100 = Unbundle By Name(w259) -> ("Command"=w258:T21, "Data"=w257:u32)
        n101 = case shown="\"Start Auto SPI\"" w258 {
          tunnel: w256 -> [w269 w274 w282 w287 w301 w310 w355]
          tunnel: w266 -> [w270 w273 w277 w285 w306 w333 w365]
          tunnel: [w270 w273 w276 w284 w306 w316 w353] -> w265
          tunnel: [w269 w272 w282 w288 w300 w309 w355] -> w264
          tunnel: w263 -> [_ _ _ _ w305 _ _]
          tunnel: w262 -> [_ _ _ w292 w303 _ _]
          tunnel: w260 -> [_ _ _ w290 _ w331 w367]
          tunnel: w257 -> [_ _ w278 _ _ _ _]
          tunnel: w256 -> [_ _ _ _ _ w330 w358]
          tunnel: w255 -> [_ _ w275 w283 _ w307 _]
          frame "None", Default {
          }
          frame "Reset" {
            n102 = Bundle By Name(cluster=w274, "Reset"=TRUE ("First Run")) -> (w272:T15)
          }
          frame "Set Calibration Period" {
            w280 = T14 102 items=["Reserved1"=0, "DIAG_STAT"=2, "X_GYRO_LOW"=4, "X_GYRO_OUT"=6, "Y_GYRO_LOW"=8, "Y_GYRO_OUT"=10, "Z_GYRO_LOW"=12, "Z_GYRO_OUT"=14, "X_ACCL_LOW"=16, "X_ACCL_OUT"=18, "Y_ACCL_LOW"=20, "Y_ACCL_OUT"=22, "Z_ACCL_LOW"=24, "Z_ACCL_OUT"=26, "TEMP_OUT"=28, "TIME_STAMP"=30, "Reseved2"=32, "DATA_CNTR"=34, "X_DELTANG_LOW"=36, "X_DELTANG_OUT"=38, "Y_DELTANG_LOW"=40, "Y_DELTANG_OUT"=42, "Z_DELTANG_LOW"=44, "Z_DELTANG_OUT"=46, "X_DELTVEL_LOW"=48, "X_DELTVEL_OUT"=50, "Y_DELTVEL_LOW"=52, "Y_DELTVEL_OUT"=54, "Z_DELTVEL_LOW"=56, "Z_DELTVEL_OUT"=58, "Reserved3"=60, "Reserved4"=62, "XG_BIAS_LOW"=64, "XG_BIAS_HIGH"=66, "YG_BIAS_LOW"=68, "YG_BIAS_OUT"=70, "ZG_BIAS_LOW"=72, "ZG_BIAS_OUT"=74, "XA_BIAS_LOW"=76, "XA_BIAS_HIGH"=78, "YA_BIAS_LOW"=80, "YA_BIAS_OUT"=82, "ZA_BIAS_LOW"=84, "ZA_BIAS_OUT"=86, "Reserved5"=88, "Reserved6"=90, "FILT_CTRL"=92, "Reserved5"=94, "MSC_CTRL"=96, "UP_SCALE"=98, "DEC_RATE"=100, "NULL_CNFG"=102, "GLOB_CMD"=104, "Reserved6"=106, "FIRM_REV"=108, "FIRM_DM"=110, "FIRM_Y"=112, "PROD_ID"=114, "SERIAL_NUM"=116, "USER_SCR1"=118, "USER_SCR2"=120, "USER_SCR3"=122, "FLSHCNT_LOW"=124, "FLSHCNT_HIGH"=126] ("Register")
            w281 = 1792  # Data
            n103 = Or(x=w278, y=w281) -> (x .or. y?=w279:u32)
            n104 = call "ADIS16470 Write Register.vi"("error in (no error)"=w277, "Data"=w279, "Register"=w280, "SPIDevRef in"=w275) -> ("error out"=w276:errorcluster)  [unwired: 6 in, 1 out]
          }
          frame "Recalibrate" {
            w293 = T14 104 items=["Reserved1"=0, "DIAG_STAT"=2, "X_GYRO_LOW"=4, "X_GYRO_OUT"=6, "Y_GYRO_LOW"=8, "Y_GYRO_OUT"=10, "Z_GYRO_LOW"=12, "Z_GYRO_OUT"=14, "X_ACCL_LOW"=16, "X_ACCL_OUT"=18, "Y_ACCL_LOW"=20, "Y_ACCL_OUT"=22, "Z_ACCL_LOW"=24, "Z_ACCL_OUT"=26, "TEMP_OUT"=28, "TIME_STAMP"=30, "Reseved2"=32, "DATA_CNTR"=34, "X_DELTANG_LOW"=36, "X_DELTANG_OUT"=38, "Y_DELTANG_LOW"=40, "Y_DELTANG_OUT"=42, "Z_DELTANG_LOW"=44, "Z_DELTANG_OUT"=46, "X_DELTVEL_LOW"=48, "X_DELTVEL_OUT"=50, "Y_DELTVEL_LOW"=52, "Y_DELTVEL_OUT"=54, "Z_DELTVEL_LOW"=56, "Z_DELTVEL_OUT"=58, "Reserved3"=60, "Reserved4"=62, "XG_BIAS_LOW"=64, "XG_BIAS_HIGH"=66, "YG_BIAS_LOW"=68, "YG_BIAS_OUT"=70, "ZG_BIAS_LOW"=72, "ZG_BIAS_OUT"=74, "XA_BIAS_LOW"=76, "XA_BIAS_HIGH"=78, "YA_BIAS_LOW"=80, "YA_BIAS_OUT"=82, "ZA_BIAS_LOW"=84, "ZA_BIAS_OUT"=86, "Reserved5"=88, "Reserved6"=90, "FILT_CTRL"=92, "Reserved5"=94, "MSC_CTRL"=96, "UP_SCALE"=98, "DEC_RATE"=100, "NULL_CNFG"=102, "GLOB_CMD"=104, "Reserved6"=106, "FIRM_REV"=108, "FIRM_DM"=110, "FIRM_Y"=112, "PROD_ID"=114, "SERIAL_NUM"=116, "USER_SCR1"=118, "USER_SCR2"=120, "USER_SCR3"=122, "FLSHCNT_LOW"=124, "FLSHCNT_HIGH"=126] ("Register")
            w296 = u16 1  # Data
            # "Write Calibration"
            # "GLOB_CMD Timing"
            n105 = RT FIFO Write(0:w292, 1:T16 {"Calibrated?"=FALSE, "IMU Detected?"=TRUE} ("element")) -> ()  [unwired: 3 in, 4 out]
            n106 = RT FIFO Write(0:w290, 1:T17 {"Command"=enum."Start Auto SPI", "Data"=0} ("element")) -> ()  [unwired: 3 in, 4 out]
            n107 = call "ADIS16470 Write Register.vi"("error in (no error)"=w285, "Data"=w296, "Register"=w293, "SPIDevRef in"=w283) -> ("error out"=w295:errorcluster, "SPIDevRef out"=w294:T13)  [unwired: 6 in]
            n108 = flat-sequence {
              tunnel: w295 -> [w298]
              tunnel: [w298] -> w284
              tunnel: w294 -> [_]
              frame #0 {
                n109 = Wait (ms)(milliseconds to wait=u32 50) -> ()  [unwired: 1 out]
              }
            }
            n110 = Bundle By Name(cluster=w287, "Reset"=TRUE) -> (w288:T15)
          }
          frame "Recal Complete" {
            n111 = Send Notification(notification="", notifier=w305) -> ()  [unwired: 1 in, 2 out]
            n112 = RT FIFO Write(0:w303, 1:T16 {"Calibrated?"=TRUE, "IMU Detected?"=TRUE} ("element")) -> ()  [unwired: 3 in, 4 out]
            n113 = Bundle By Name(cluster=w301, "AutoSPI Active?"=TRUE) -> (w300:T15)
          }
          frame "Exit Auto SPI" {
            w326 = T14 114 items=["Reserved1"=0, "DIAG_STAT"=2, "X_GYRO_LOW"=4, "X_GYRO_OUT"=6, "Y_GYRO_LOW"=8, "Y_GYRO_OUT"=10, "Z_GYRO_LOW"=12, "Z_GYRO_OUT"=14, "X_ACCL_LOW"=16, "X_ACCL_OUT"=18, "Y_ACCL_LOW"=20, "Y_ACCL_OUT"=22, "Z_ACCL_LOW"=24, "Z_ACCL_OUT"=26, "TEMP_OUT"=28, "TIME_STAMP"=30, "Reseved2"=32, "DATA_CNTR"=34, "X_DELTANG_LOW"=36, "X_DELTANG_OUT"=38, "Y_DELTANG_LOW"=40, "Y_DELTANG_OUT"=42, "Z_DELTANG_LOW"=44, "Z_DELTANG_OUT"=46, "X_DELTVEL_LOW"=48, "X_DELTVEL_OUT"=50, "Y_DELTVEL_LOW"=52, "Y_DELTVEL_OUT"=54, "Z_DELTVEL_LOW"=56, "Z_DELTVEL_OUT"=58, "Reserved3"=60, "Reserved4"=62, "XG_BIAS_LOW"=64, "XG_BIAS_HIGH"=66, "YG_BIAS_LOW"=68, "YG_BIAS_OUT"=70, "ZG_BIAS_LOW"=72, "ZG_BIAS_OUT"=74, "XA_BIAS_LOW"=76, "XA_BIAS_HIGH"=78, "YA_BIAS_LOW"=80, "YA_BIAS_OUT"=82, "ZA_BIAS_LOW"=84, "ZA_BIAS_OUT"=86, "Reserved5"=88, "Reserved6"=90, "FILT_CTRL"=92, "Reserved5"=94, "MSC_CTRL"=96, "UP_SCALE"=98, "DEC_RATE"=100, "NULL_CNFG"=102, "GLOB_CMD"=104, "Reserved6"=106, "FIRM_REV"=108, "FIRM_DM"=110, "FIRM_Y"=112, "PROD_ID"=114, "SERIAL_NUM"=116, "USER_SCR1"=118, "USER_SCR2"=120, "USER_SCR3"=122, "FLSHCNT_LOW"=124, "FLSHCNT_HIGH"=126] ("ADIS16448 Register")
            n114 = Unbundle By Name(w330) -> ("ADIS16470DevRef.Hardware Config.IMU SPI Bus"=w329:T7, "ADIS16470DevRef.Hardware Config.SPI Clock Rate (Hz)"=w328:dbl, "ADIS16470DevRef.Hardware Config.IMU SPI Mode (3)"=w327:T5)
            n115 = call <vilib>:"WPI_SPIClose.vi"("error in (no error)"=w333, "SPIDevRef"=w307) -> ("error out"=w312:errorcluster)  [unwired: 9 in]
            n116 = call <vilib>:"WPI_DigitalOutputRefNum Registry Get.vi"("error in (no error)"=w312, "refnum name"="470 Status LED") -> ("error out"=w314:errorcluster, "DigitalOutputDevRef"=w313:T18)  [unwired: 8 in]
            n117 = call <vilib>:"WPI_DigitalOutputSetValue.vi"("error in (no error)"=w314, "Value"=TRUE, "DigitalOutputDevRef"=w313) -> ("error out"=w311:errorcluster)  [unwired: 7 in, 1 out]
            n118 = RT FIFO Write(0:w331, 1:T17 {"Command"=enum."Recalibrate", "Data"=0} ("element")) -> ()  [unwired: 3 in, 4 out]
            n119 = call <vilib>:"WPI_SPIOpen.vi"("error in"=w311, "Mode (3)"=w327, "Clock Rate (Hz)"=w328, "SPI Bus"=w329) -> ("error out"=w325:errorcluster, "SPIDevRef"=w318:T13)  [unwired: 6 in]
            n120 = call "ADIS16470 Read Register.vi"("error in (no error)"=w325, "ADIS16470 Register"=w326, "SPIDevRef in"=w318) -> ("error out"=w319:errorcluster, "Register Value"=w317:u16, "SPIDevRef out"=w320:T13)  [unwired: 6 in]
            n121 = Or(x=u16 16982 ("y"), y=u16 16470) -> (x .or. y?=w322:u16)
            n122 = Equal?(x=w322, y=w317) -> (x = y?=w321:bool)
            n123 = case shown="True" w321 {
              tunnel: w320 -> [_ w347]
              tunnel: w319 -> [w336 w346]
              tunnel: [w335 w345] -> w316
              tunnel: w310 -> [w334 w343]
              tunnel: [w334 w342] -> w309
              frame False {
                n124 = case shown="No Error" w336 {
                  selector: w336 -> [w338 w341]
                  tunnel: [w337 w341] -> w335
                  frame No Error {
                    n125 = call <vilib>:"Error Cluster From Error Code.vi"("error in (no error)"=w338, "error message (\"\")"="SPI port did not reset properly" ("error message (\"\")"), "error code (0)"=-8106) -> ("error out"=w337:errorcluster)  [unwired: 6 in]
                  }
                  frame Error {
                  }
                }
              }
              frame True {
                n126 = call <vilib>:"WPI_SPIRefNum Registry Set.vi"("error in (no error)"=w346, "refnum name"="AutoSPI", "SPIDevRef"=w347) -> ("error out"=w345:errorcluster, "SPIDevRef"=w348:T13)  [unwired: 7 in]
                n127 = Bundle By Name(cluster=w343, "SPIDevRef"=w348, "AutoSPI Active?"=FALSE) -> (w342:T15)
              }
            }
          }
          frame "Start Auto SPI" {
            n128 = Unbundle By Name(w358) -> ("Digital Source"=w357:T9, "SPIDevRef.SPI Bus"=w352:T7, "ADIS16470DevRef.Hardware Config.Stall Config"=w351:T20, "Data Packet"=w350:T14[])
            n129 = RT FIFO Write(0:w367, 1:T17 {"Command"=enum."Recal Complete", "Data"=0} ("element")) -> ()  [unwired: 3 in, 4 out]
            n130 = call <vilib>:"FPGA_SPI_ConfigureAuto.vi"("SPI Auto Zero Byte Count"=u8 0, "error in"=w365, "SPI Auto TX Byte Array"=w350, "Stall Config"=w351, "SPI Bus"=w352) -> ("error out"=w356:errorcluster)  [unwired: 6 in]
            n131 = call <vilib>:"FPGA_SPI_StartAuto_External.vi"("error in (no error)"=w356, "Falling Edge"=FALSE, "Rising Edge"=TRUE, "Source"=w357) -> ("error out"=w362:errorcluster)  [unwired: 7 in]
            n132 = call <vilib>:"WPI_DigitalOutputRefNum Registry Get.vi"("error in (no error)"=w362, "refnum name"="470 Status LED") -> ("error out"=w361:errorcluster, "DigitalOutputDevRef"=w360:T18)  [unwired: 8 in]
            n133 = call <vilib>:"WPI_DigitalOutputSetValue.vi"("error in (no error)"=w361, "Value"=FALSE, "DigitalOutputDevRef"=w360) -> ("error out"=w353:errorcluster)  [unwired: 7 in, 1 out]
          }
        }
      }
    }
  }
  n134 = while {
    tunnel: w8 -> [w370]
    tunnel: [w369] -> w2
    stop <- w369 stop-if-true
    # "stop this VI when the VI calling StartComm goes idle"
    n135 = property class="VI"(reference=w370) -> ("Exec.State"=w372:T22)  [unwired: 1 in, 2 out]
    n136 = Wait (ms)(milliseconds to wait=u32 250) -> ()  [unwired: 1 out]
    n137 = Equal?(x=w372, y=T22."Idle" ("Execution:State")) -> (x = y?=w369:bool)
  }
  n138 = flat-sequence {
    tunnel: w2 -> [_]
    frame #0 {
      n139 = call <vilib>:"WPI_DigitalOutputRefNum Registry Get.vi"("refnum name"="470 Status LED") -> ("error out"=w383:errorcluster, "DigitalOutputDevRef"=w382:T18)  [unwired: 9 in]
      n140 = call <vilib>:"WPI_DigitalOutputClose.vi"("error in (no error)"=w383, "DigitalOutputDevRef"=w382) -> ("error out"=w381:errorcluster)  [unwired: 9 in]
      n141 = call <vilib>:"WPI_DigitalOutputRefNum Registry Get.vi"("error in (no error)"=w381, "refnum name"="470 Reset Pin") -> ("error out"=w379:errorcluster, "DigitalOutputDevRef"=w378:T18)  [unwired: 8 in]
      n142 = call <vilib>:"WPI_DigitalOutputClose.vi"("error in (no error)"=w379, "DigitalOutputDevRef"=w378) -> ("error out"=w377:errorcluster)  [unwired: 9 in]
      n143 = call <vilib>:"WPI_SPIRefNum Registry Get.vi"("error in (no error)"=w377, "refnum name"="AutoSPI") -> ("error out"=w375:errorcluster, "SPIDevRef"=w374:T13)  [unwired: 8 in]
      n144 = call <vilib>:"WPI_SPIClose.vi"("error in (no error)"=w375, "SPIDevRef"=w374) -> ()  [unwired: 9 in, 1 out]
    }
    frame #1 {
      n145 = Stop() -> ()  [unwired: 1 in]
    }
  }
